vi "Mutex Init.vi"(8 "error in (no error)":errorcluster, 10 "Mutex Attr in":T2, 11 "Mutex in":T1) -> (0 "error out":errorcluster, 2 "Mutex Attr out":T2, 3 "Mutex out":T1)   [LabVIEW 2013, in "Linux RT IPC.POSIX Threads.lvlib" / "Mutex.lvclass"]
doc: "Calls pthread_mutex_init() on the pthread mutex object encapsulated by Mutex.\n\nThis VI initializes the mutex object and sets its attributes using the attributes contained in the Mutex Attr object.\n\nRefer to online POSIX documentation for more information."
uses:
  Mutex.lvclass
  Controls/reference.ctl
  Mutex Attr/Controls/reference.ctl
  Mutex Attr/Mutex Attr.lvclass
  POSIX Thread Object/POSIX Thread Object.lvclass/POSIX Thread Object.ctl
  POSIX Thread Object/Private VIs/libpthread path.vi
  POSIX Thread Object/Private VIs/get pthread error.vi
  POSIX Thread Object/POSIX Thread Object.lvclass
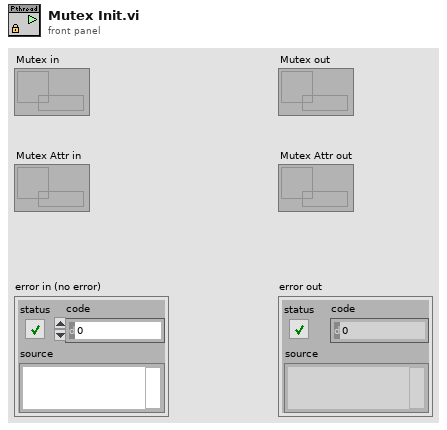
[diagram p1: front panel]
types:
  T1 = typedef "Linux RT IPC.POSIX Threads.lvlib/Mutex.lvclass/reference.ctl" = refnum<data-value>
  T2 = typedef "Linux RT IPC.POSIX Threads.lvlib/Mutex Attr.lvclass/reference.ctl" = refnum<data-value>
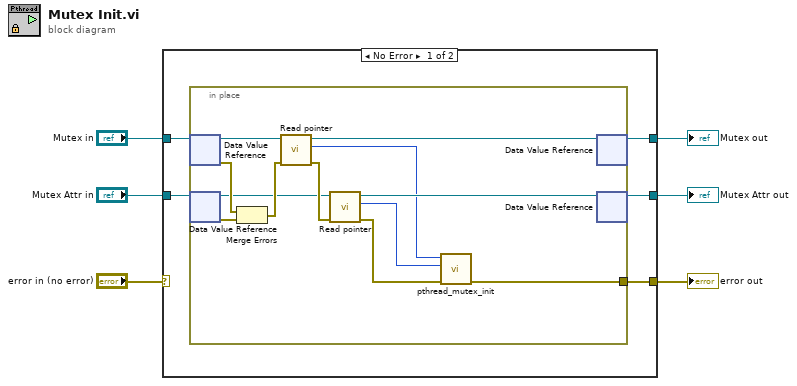
[diagram p0: block diagram]
diagram:
  n1 = case shown="No Error" "error in (no error)" {
    selector: "error in (no error)" -> [_ w26]
    tunnel: [w9 w26] -> w6
    tunnel: [w11 w25] -> w5
    tunnel: [w10 w24] -> w4
    tunnel: "Mutex Attr in" -> [w8 w24]
    tunnel: "Mutex in" -> [w7 w25]
    frame No Error {
      n2 = in-place {
        in-place-border: [w15] -> w9
        n3 = in-place-dvr #1(w7) -> (w23:refnum<class "Mutex.lvclass">, w20:errorcluster)
        n4 = in-place-dvr #2(w8) -> (w16:refnum<class "Mutex Attr.lvclass">, w21:errorcluster)
        n5 = Merge Errors(w20, w21) -> (w19:errorcluster)
        n6 = call "Read pointer.vi"("error in (no error)"=w19, "POSIX Thread Object in"=w23) -> ("error out"=w18:errorcluster, "pointer"=w12:u64, "POSIX Thread Object out"=w22:refnum<class "Mutex.lvclass">)  [unwired: 7 in]
        n7 = call "Read pointer.vi"("error in (no error)"=w18, "POSIX Thread Object in"=w16) -> ("error out"=w14:errorcluster, "pointer"=w13:u64, "POSIX Thread Object out"=w17:refnum<class "Mutex Attr.lvclass">)  [unwired: 7 in]
        n8 = call "pthread_mutex_init.vi"("error in (no error)"=w14, "mutex attr ptr in"=w13, "mutex ptr in"=w12) -> ("error out"=w15:errorcluster)  [unwired: 6 in, 2 out]
        n9 = in-place-dvr #1(w22) -> (w11:T1)  [unwired: 1 out]
        n10 = in-place-dvr #2(w17) -> (w10:T2)  [unwired: 1 out]
      }
    }
    frame Error {
    }
  }
  "Mutex out" <- w5
  "error out" <- w6
  "Mutex Attr out" <- w4
